vi "niFPGA Discrete PID.vi"(0 "setpoint":i16, 2 "process variable":i16, 3 "PID gains (x 2^8)":T1={"proportional gain (Kc)"=1, "integral gain (Kc*Ts/Ti)"=0, "derivative gain (Kc*Td/Ts)"=0}, 4 "output range":cluster{"output high":i16, "output low":i16}={"output high"=32767, "output low"=-32768}, 5 "initialize":bool) -> (7 "output":i16)   [LabVIEW 2020]
doc: "The LabVIEW FPGA Module no longer supports this VI. Use the PID (FPGA) Express VI instead. The PID (FPGA) Express VI is available with the LabVIEW PID Control toolkit.\n\nImplements an integer PID algorithm for simple PID applications or high-speed control applications that require an efficient algorithm. The PID algorithm features control output range limiting with integrator anti-windup. The PID algorithm also features bumpless controller output for PID gain changes.\n\nThe Discrete PID VI uses saturation arithmetic and internal scaling to avoid integer overflow. All scaling rounds to negative infinity.\n\nCompute the <B>PID gains (x 2^8)</B> inputs before you pass them into an FPGA VI. You can compute the required integer gain values in a host VI and pass them to a PID loop running on the FPGA target."
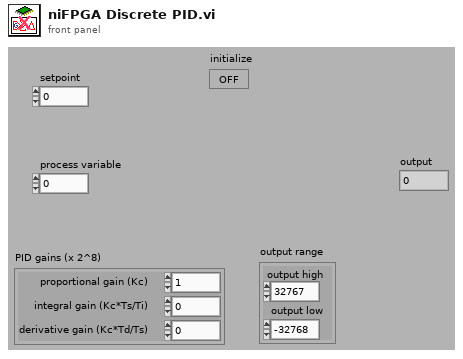
[diagram p1: front panel]
types:
  T1 = cluster{"proportional gain (Kc)":i16, "integral gain (Kc*Ts/Ti)":i16, "derivative gain (Kc*Td/Ts)":i16}
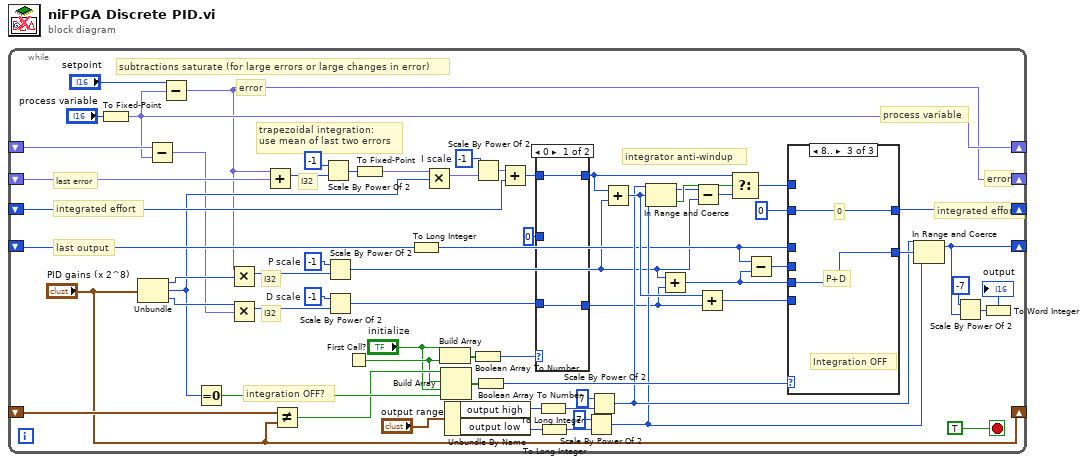
[diagram p0: block diagram]
diagram:
  n1 = while {
    shift-right: [w6] -> _
    shift-left: _ -> [w33]
    shift-right: [w14] -> _
    shift-left: _ -> [w50]
    shift-right: [w5] -> _
    shift-left: _ -> [w32]
    shift-right: [w64] -> _
    shift-left: _ -> [w63]
    shift-right: ["PID gains (x 2^8)"] -> _
    shift-left: _ -> [w62]
    stop <- TRUE stop-if-true
    w56 = i8 -1  # I scale
    w60 = i8 -1  # D scale
    w61 = i8 -1  # P scale
    # "I32"
    # "I32"
    # "I32"
    # "integration OFF?"
    # "integrator anti-windup"
    # "last output"
    # "integrated effort"
    # "trapezoidal integration:\nuse mean of last two errors"
    # "error"
    # "subtractions saturate (for large errors or large changes in error)"
    # "last error"
    # "error"
    # "process variable"
    # "integrated effort"
    n2 = To Fixed-Point(number="process variable") -> (fixed-point=w6:fxp<+/-,16,16>)  [unwired: 1 in]
    n3 = Unbundle("PID gains (x 2^8)") -> ("proportional gain (Kc)"=w28:i16, "integral gain (Kc*Ts/Ti)"=w9:i16, "derivative gain (Kc*Td/Ts)"=w26:i16)
    n4 = Subtract(x=w33, y=w6) -> (x-y=w4:fxp<+/-,16,16>)
    n5 = Subtract(x="setpoint", y=w6) -> (x-y=w5:fxp<+/-,16,16>)
    n6 = Equal To 0?(x=w9) -> (x = 0?=w54:bool)
    n7 = Multiply(x=w5, y=w28) -> (x*y=w27:i32)
    n8 = Multiply(x=w26, y=w4) -> (x*y=w25:i32)
    n9 = Add(x=w5, y=w32) -> (x+y=w31:i32)
    n10 = Not Equal?(x=w62, y="PID gains (x 2^8)") -> (x != y?=w12:bool)
    n11 = Scale By Power Of 2(n=i8 -1, x=w31) -> (x*2^n=w58:i32)
    n12 = Scale By Power Of 2(n=w61, x=w27) -> (x*2^n=w2:i32)
    n13 = Scale By Power Of 2(n=w60, x=w25) -> (x*2^n=w1:i32)
    n14 = First Call?() -> (First Call?: T/F=w11:bool)
    n15 = To Fixed-Point(number=w58) -> (fixed-point=w30:fxp<+/-,16,16>)  [unwired: 1 in]
    n16 = To Long Integer(number=w50) -> (32bit integer=w8:i32)
    n17 = Multiply(x=w30, y=w9) -> (x*y=w29:fxp<+/-,32,32>)
    n18 = Build Array("initialize", w11) -> (w38:bool[])
    n19 = Build Array(w12, w11, "initialize", w54) -> (w53:bool[])
    n20 = Unbundle By Name("output range") -> ("output high"=w42:i16, "output low"=w20:i16)
    n21 = Scale By Power Of 2(n=w56, x=w29) -> (x*2^n=w55:fxp<+/-,32,32>)
    n22 = Boolean Array To Number(Boolean array=w38) -> (number=w37:u8)
    n23 = Boolean Array To Number(Boolean array=w53) -> (number=w52:u8)
    n24 = Add(x=w55, y=w63) -> (x+y=w36:i32)
    n25 = case shown="0" w37 {
      tunnel: w36 -> [w66 _]
      tunnel: w1 -> [w67 _]
      tunnel: [w67 w68] -> w13
      tunnel: [w66 w68] -> w35
      tunnel: 0 ("t") -> [_ w68]
      frame 0 {
      }
      frame Default {
        # "Init/\nFirst call"
      }
    }
    n26 = To Long Integer(number=w42) -> (32bit integer=w22:i32)
    n27 = To Long Integer(number=w20) -> (32bit integer=w19:i32)
    n28 = Scale By Power Of 2(n=7, x=w19) -> (x*2^n=w18:i32)
    n29 = Scale By Power Of 2(n=7, x=w22) -> (x*2^n=w24:i32)
    n30 = Add(x=w35, y=w2) -> (x+y=w44:i32)
    n31 = In Range and Coerce(upper limit=w24, x=w44, lower limit=w18) -> (coerced(x)=w43:i32, In Range?=w45:bool)
    n32 = Add(x=w2, y=w13) -> (x+y=w49:i32)
    n33 = Subtract(x=w43, y=w2) -> (x-y=w46:i32)
    n34 = Add(x=w44, y=w13) -> (x+y=w41:i32)
    n35 = Select(t=w35, s=w45, f=w46) -> (s? t:f=w40:i32)
    n36 = Subtract(x=w8, y=w49) -> (x-y=w48:i32)
    n37 = case shown="8.." w52 {
      tunnel: [w69 w72 w73] -> w64
      tunnel: [w70 w71 w74] -> w51
      tunnel: w49 -> [_ _ w74]
      tunnel: w48 -> [_ w72 _]
      tunnel: w41 -> [w70 _ _]
      tunnel: w40 -> [w69 _ _]
      tunnel: w8 -> [_ w71 _]
      tunnel: 0 ("t") -> [_ _ w73]
      frame Default {
        # "normal PID\nor\nInit/First call\nw/ integration ON"
      }
      frame 1 {
        # "last output - (P+D)"
        # "last output"
        # "PID gains have \nchanged since last iteration"
        # "P+D"
      }
      frame 8.. {
        # "0"
        # "P+D"
        # "Integration OFF"
      }
    }
    n38 = In Range and Coerce(upper limit=w24, x=w51, lower limit=w18) -> (coerced(x)=w14:i32)  [unwired: 1 out]
    n39 = Scale By Power Of 2(n=-7, x=w14) -> (x*2^n=w16:i32)
    n40 = To Word Integer(number=w16) -> (16bit integer=→"output":i16)
  }
